vi "axex_get_sheet_names.vi"(8 "error in":errorcluster, 11 "AX Excel instance in":T1) -> (0 "error out":errorcluster, 1 "sheets count":i32, 2 "sheet names":string[](array[string]), 3 "AX Excel instance out":T1, 4 "sheet tab colors":u32[](array[colorbox]))   [LabVIEW 2020, in "AX Excel.lvlib"]
doc: "Call this to obtain sheet names and count within given excel file."
uses:
  AX Excel.lvlib
  axex_instance.ctl
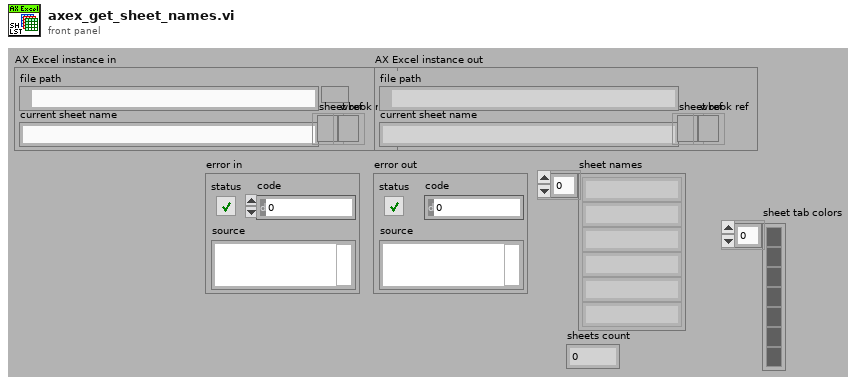
[diagram p1: front panel]
types:
  T1 = typedef "AX Excel.lvlib/axex_instance.ctl" = cluster{"file path":path, "current sheet name":string, "sheet ref":refnum<k7>, "wbook ref":refnum<k7>}
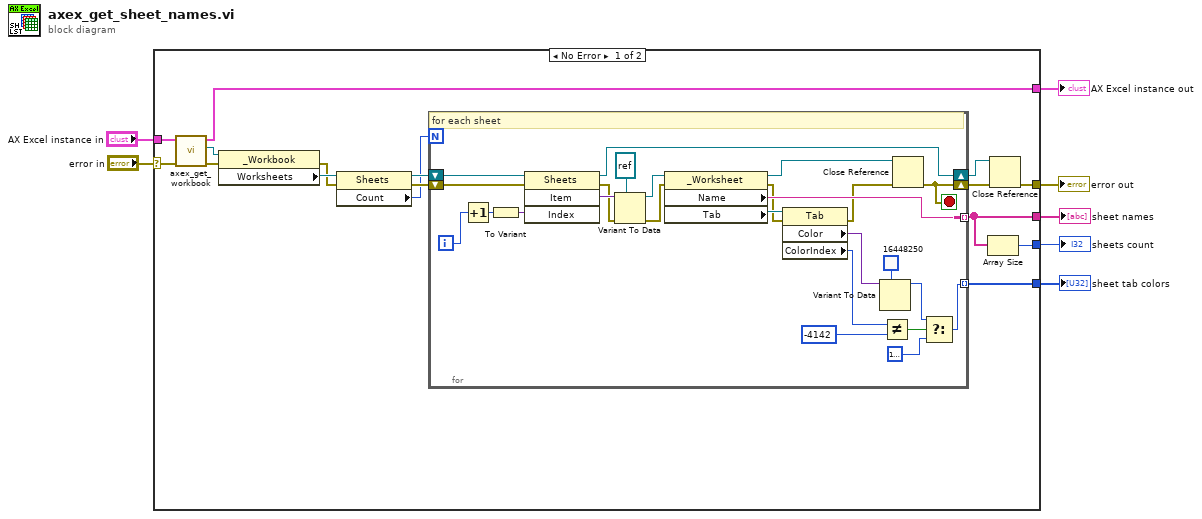
[diagram p0: block diagram]
diagram:
  n1 = case shown="No Error" "error in" {
    selector: "error in" -> [w9 w49]
    tunnel: [w15 _] -> w7
    tunnel: [w14 _] -> w6
    tunnel: "AX Excel instance in" -> [w13 w50]
    tunnel: [w11 w50] -> w4
    tunnel: [w10 w49] -> w3
    tunnel: [w8 _] -> w1
    frame No Error {
      n2 = call "axex_get_workbook.vi"("error in"=w9, "AX Excel instance in"=w13) -> ("error out"=w23:errorcluster, "excel workbook"=w12:refnum<k7>, "AX Excel instance out"=w11:T1)  [unwired: 7 in]
      n3 = property class="_Workbook"(reference=w12, error in=w23) -> (error out=w21:errorcluster, "Worksheets"=w22:refnum<k7>)  [unwired: 1 out]
      n4 = property class="Sheets"(reference=w22, error in=w21) -> (reference out=w20:refnum<k7>, error out=w19:errorcluster, "Count"=w18:i32)
      n5 = for {
        N: w18 -> [_]
        shift-right: [w36] -> w17
        shift-left: w19 -> [w45]
        tunnel: [w38] -> w15 mode=indexing
        shift-right: [w35] -> w16
        shift-left: w20 -> [w37]
        tunnel: [w26] -> w8 mode=indexing
        i -> [w46]
        stop <- w36 stop-if-true
        # "for each sheet"
        n6 = Increment(x=w46) -> (x+1=w47:i32)
        n7 = To Variant(anything=w47) -> (Variant=w48:variant)
        n8 = invoke class="Sheets" method="Item"(reference=w37, error in=w45, "Index"=w48) -> (reference out=w35:refnum<k7>, error out=w41:errorcluster, "Item"=w44:variant)  [unwired: 1 in, 1 out]
        n9 = Variant To Data(error in=w41, type=refnum<k7> refnum ("reference out"), Variant=w44) -> (data=w42:refnum<k7>, error out=w40:errorcluster)
        n10 = property class="_Worksheet"(reference=w42, error in=w40) -> (reference out=w39:refnum<k7>, error out=w25:errorcluster, "Name"=w38:string, "Tab"=w34:refnum<k7>)
        n11 = property class="Tab"(reference=w34, error in=w25) -> (error out=w24:errorcluster, "Color"=w32:variant, "ColorIndex"=w30:i32)  [unwired: 1 out]
        n12 = Variant To Data(type=u32 16448250, Variant=w32) -> (data=w28:u32)  [unwired: 1 in, 1 out]
        n13 = Not Equal?(x=w30, y=-4142) -> (x != y?=w29:bool)
        n14 = Close Reference(reference=w39, error in (no error)=w24) -> (error out=w36:errorcluster)
        n15 = Select(t=w28, s=w29, f=u32 16777216) -> (s? t:f=w26:u32)
      }
      n16 = Array Size(array=w15) -> (size(s)=w14:i32)
      n17 = Close Reference(reference=w16, error in (no error)=w17) -> (error out=w10:errorcluster)
    }
    frame Error {
    }
  }
  "error out" <- w3
  "sheet names" <- w7
  "sheets count" <- w6
  "AX Excel instance out" <- w4
  "sheet tab colors" <- w1
